vi "题目一的子vi.vi"() -> ()   [LabVIEW 2017]
panel:
  in  "滑动杆":i32(slide) scale=0.0..10.0
  out "波形图表":dbl[](graph)
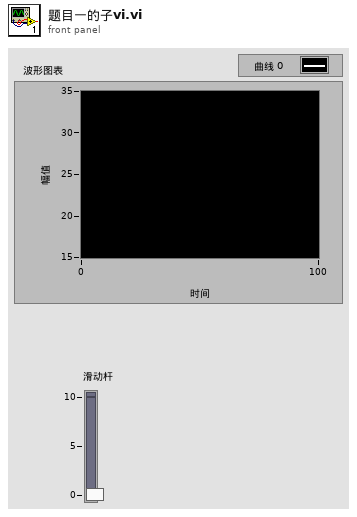
[diagram p1: front panel]
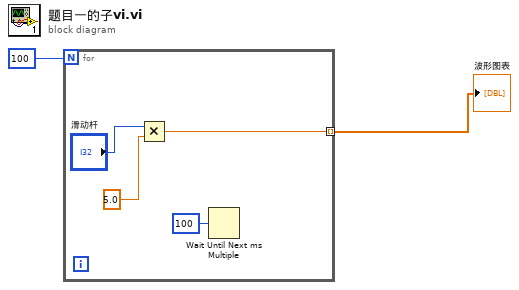
[diagram p0: block diagram]
diagram:
  n1 = for {
    N: 100 -> [_]
    tunnel: [w5] -> w1 mode=indexing
    n2 = Multiply(x="滑动杆", y=5.0) -> (x*y=w5:dbl)
    n3 = Wait Until Next ms Multiple(millisecond multiple=u32 100 ("毫秒倍数")) -> ()  [unwired: 1 out]
  }
  "波形图表" <- w1
